vi "TP 1.6 (SubVI).vi"(1 "Temp inicial":dbl) -> (0 "Numeric":dbl)   [LabVIEW 2013]
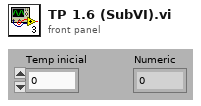
[diagram p1: front panel]
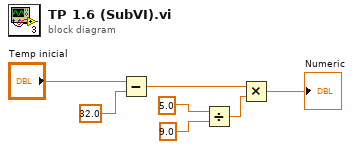
[diagram p0: block diagram]
diagram:
  n1 = Subtract(x="Temp inicial", y=32.0) -> (x-y=w3:dbl)
  n2 = Divide(x=5.0 ("x/y"), y=9.0 ("x/y")) -> (x/y=w4:dbl)
  n3 = Multiply(x=w3, y=w4) -> (x*y=→"Numeric":dbl)
